vi "Repeat.vi"(1 "Iterations":i32, 2 "Script":string="pump /1Q #query pump\npump /1? #report absolute plunger position\npump /1?6 #report valve position") -> (0 "Output":string)   [LabVIEW 2019]
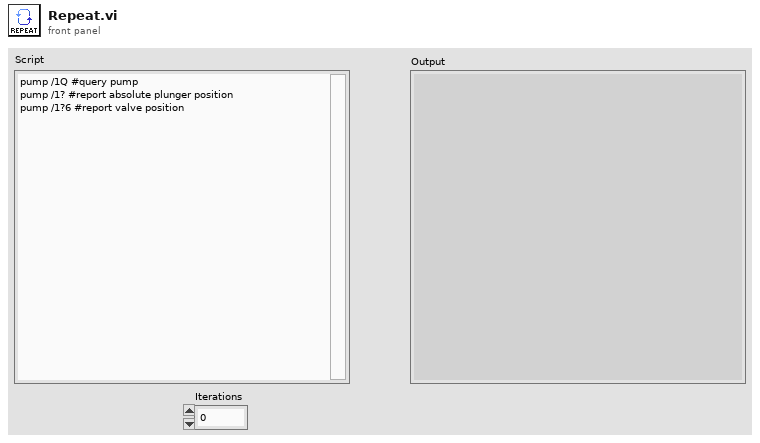
[diagram p1: front panel]
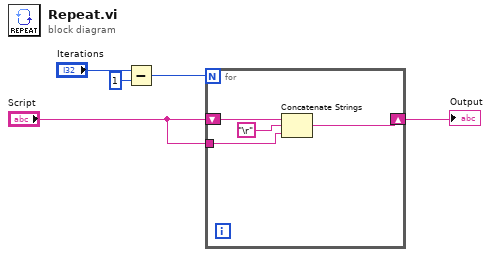
[diagram p0: block diagram]
diagram:
  n1 = Subtract(x="Iterations", y=1) -> (x-y=w2:i32)
  n2 = for {
    N: w2 -> [_]
    shift-right: [w8] -> w5
    shift-left: "Script" -> [w9]
    tunnel: "Script" -> [w6]
    n3 = Concatenate Strings(w9, "\r", w6) -> (w8:string)
  }
  "Output" <- w5
